vi "读用户名.vi"(2 "error in (no error)":errorcluster) -> (0 "error out":errorcluster, 1 "SQL Results":string[][](table))   [LabVIEW 2013]
doc: "This example opens a connection to a database specified by the Connection string (replace the DNS name with your database) and retrieves all the rows and columns from the table \"Table1\" (replace the SQL string with your own SQL query)."
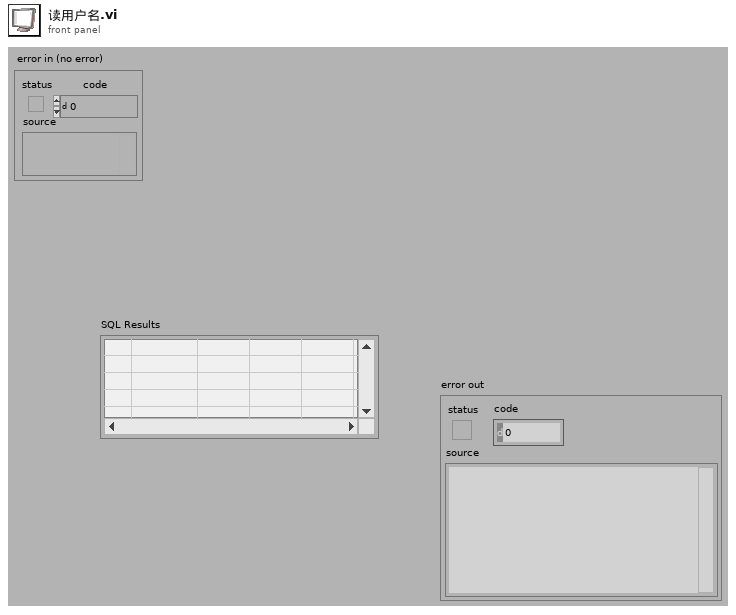
[diagram p1: front panel]
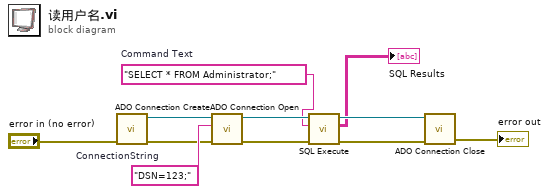
[diagram p0: block diagram]
diagram:
  w6 = "SELECT * FROM Administrator;"  # Command Text
  w4 = "DSN=123;"  # ConnectionString
  n1 = call <nishared>:"ADO Connection Create.vi"("error in (no error)"="error in (no error)") -> ("error out"=w3:errorcluster, "ADODB._Connection Out"=w2:refnum<k7>)  [unwired: 9 in]
  n2 = call <nishared>:"ADO Connection Open.vi"("error in (no error)"=w3, "ConnectionString"=w4, "ADODB._Connection In"=w2) -> ("error out"=w9:errorcluster, "ADODB._Connection Out"=w10:refnum<k7>)  [unwired: 7 in]
  n3 = call <nishared>:"SQL Execute.vi"("error in (no error)"=w9, "Command Text"=w6, "ADODB._Connection In"=w10) -> ("error out"=w8:errorcluster, "Data"=→"SQL Results":string[][], "ADODB._Connection Out"=w11:refnum<k7>)  [unwired: 5 in, 1 out]
  n4 = call <nishared>:"ADO Connection Close.vi"("error in (no error)"=w8, "ADODB._Connection In"=w11) -> ("error out"=→"error out":errorcluster)  [unwired: 8 in, 1 out]
